vi "Open_RESTful_connection.vi"(8 "error in (no error)":errorcluster) -> (0 "error out":errorcluster, 3 "REST Client out":refnum<class "REST Client.lvclass">)   [LabVIEW 2024]
uses:
  <vilib>/addons/_JKI.lib/REST Client/classes/REST Client/REST Client.lvclass
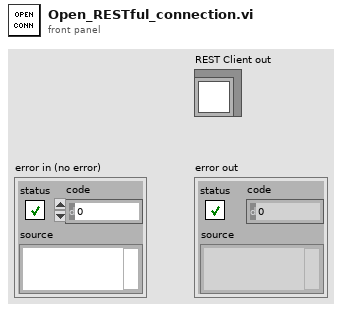
[diagram p1: front panel]
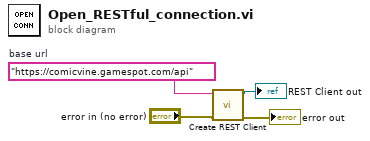
[diagram p0: block diagram]
diagram:
  w4 = "https://comicvine.gamespot.com/api"  # base url
  n1 = call <vilib>:"Create REST Client.vi"("error in (no error)"="error in (no error)", "Base URL"=w4) -> ("error out"=→"error out":errorcluster, "REST Client out"=→"REST Client out":refnum<class "REST Client.lvclass">)  [unwired: 8 in]
